vi "US fuel price.vi"() -> ()   [LabVIEW 2023]
doc: "Converts UK Fuel Prices to US fuel prices and vice versa"
panel:
  out "How much more expensive UK fuel is than US fuel":dbl=65.88302868943256 format="%#.1f %"
  out "How much cheaper US fuel is compared to UK fuel":dbl=63.12732642953957 format="%#.1g %"
  in  "stop":bool
  out "Price of UK Fuel converted to US units":dbl=7.079219668874475 format="$%02.2f/Gallon (US)"
  in  "Price of Fuel In US":dbl=3.39 format="$%02.2f/Gallon (US)"
  out "Price of US fuel converted to UK units":dbl=0.68956752697803 format="£%02.2f/Litre (UK)"
  in  "Dollar exchange rate":dbl=0.77 format="£%02.2f /$"
  in  "Price of Fuel In UK":dbl=1.44 format="£%02.2f/Litre (UK)"
  # "US-UK Fuel Price Convertor"
  # "Instructions\n1) Look up US dollar exchange rate (https://www.xe.com/en-gb/currencyconverter/convert/?Amount=1&From=USD&To=GBP) and update\n\n2) Look up UK fuel price (https://www.rac.co.uk/drive/advice/fuel-watch/) and update\n\n3) Look up US fuel price (https://gasprices.aaa.com/) and update\n\n4) Observe calculated values"
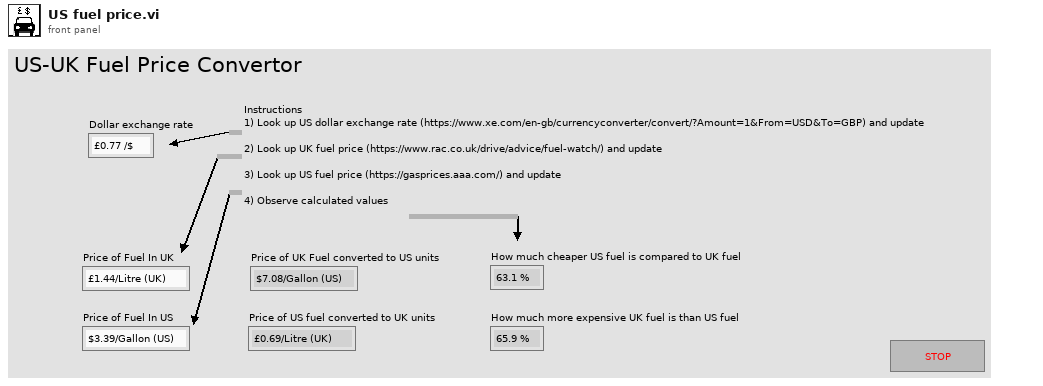
[diagram p1: front panel]
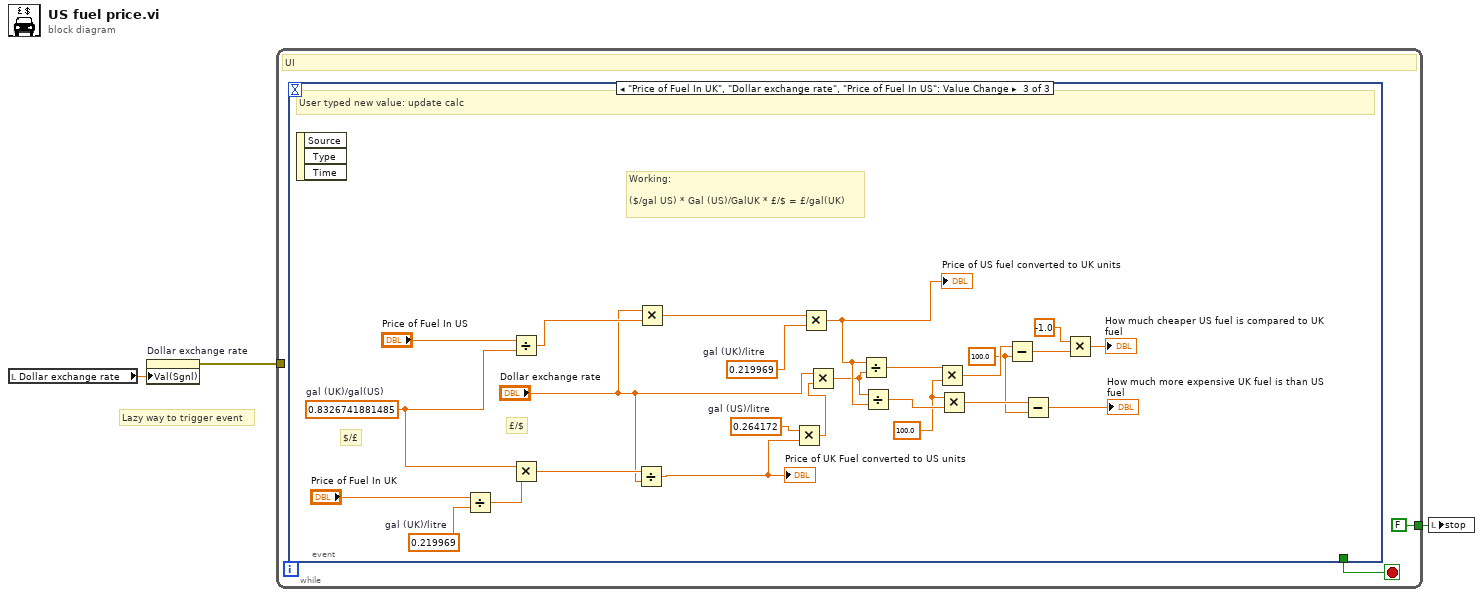
[diagram p0: block diagram]
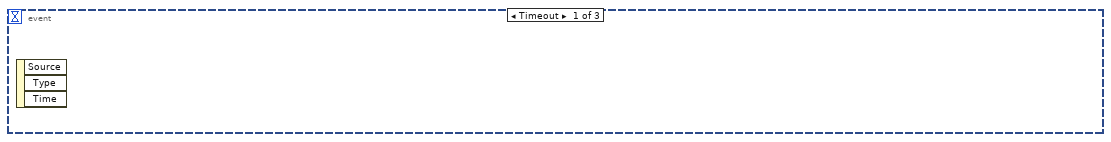
[diagram p2: hidden frame]
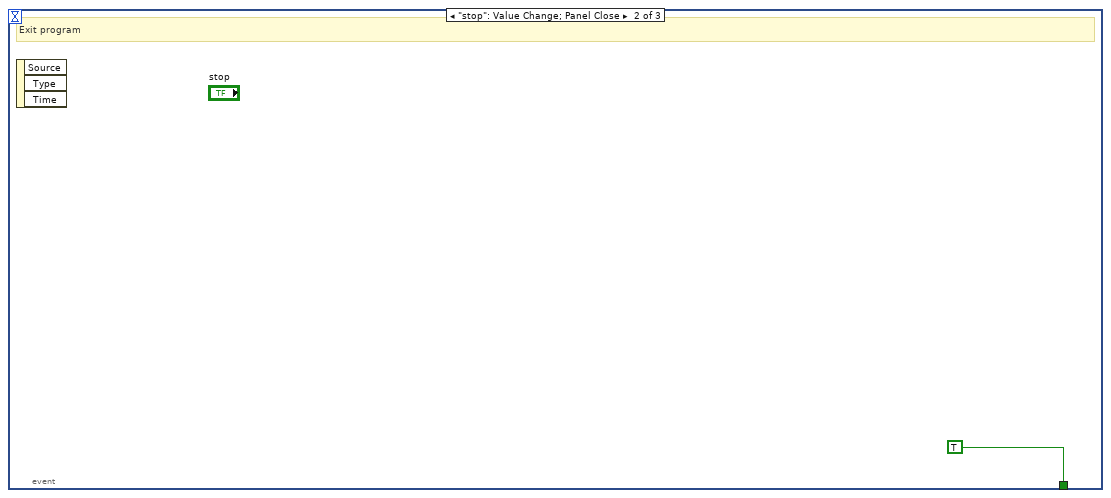
[diagram p3: hidden frame]
diagram:
  # "Lazy way to trigger event"
  n1 = local read "Dollar exchange rate"() -> (w2:dbl)
  n2 = property on="Dollar exchange rate" class="DigNum (strict)"("Val(Sgnl)"=w2) -> (error out=w1:errorcluster)  [unwired: 2 in, 1 out]
  n3 = while {
    tunnel: [FALSE ("stop")] -> w3
    tunnel: w1 -> [_]
    stop <- w5 stop-if-true
    # "UI"
    n4 = event shown="[2] \"Price of Fuel In UK\", \"Dollar exchange rate\", \"Price of Fuel In US\": Value Change" {
      selector: _ -> [_ _ _]
      dyn-events: _ -> [_ _ _]
      timeout: _ -> [_ _ _]
      tunnel: [_ TRUE _] -> w5
      event Timeout {
        n5 = event-data() -> ()  [unwired: 1 in, 3 out]
      }
      event "stop": Value Change; Panel Close {
        # "Exit program"
        n6 = event-data() -> ()  [unwired: 1 in, 3 out]
      }
      event "Price of Fuel In UK", "Dollar exchange rate", "Price of Fuel In US": Value Change {
        w15 = 100.0 ("y")
        w14 = 100.0 ("y")
        w13 = 0.264172  # gal (US)/litre
        w12 = 0.219969  # gal (UK)/litre
        w11 = 0.219969  # gal (UK)/litre
        w10 = 0.8326741881485  # gal (UK)/gal(US)
        # "Working:\n\n($/gal US) * Gal (US)/GalUK * £/$ = £/gal(UK)"
        # "£/$"
        # "$/£"
        # "User typed new value: update calc"
        n7 = event-data() -> ()  [unwired: 1 in, 3 out]
        n8 = Divide(x="Price of Fuel In UK", y=w12) -> (x/y=w22:dbl)
        n9 = Divide(x="Price of Fuel In US", y=w10) -> (x/y=w19:dbl)
        n10 = Multiply(x=w10, y=w22) -> (x*y=w18:dbl)
        n11 = Divide(x=w18, y="Dollar exchange rate") -> (x/y=w23:dbl)
        "Price of UK Fuel converted to US units" <- w23
        n12 = Multiply(x="Dollar exchange rate", y=w19) -> (x*y=w20:dbl)
        n13 = Multiply(x=w13, y=w23) -> (x*y=w9:dbl)
        n14 = Multiply(x=w20, y=w11) -> (x*y=w24:dbl)
        "Price of US fuel converted to UK units" <- w24
        n15 = Multiply(x="Dollar exchange rate", y=w9) -> (x*y=w7:dbl)
        n16 = Divide(x=w24, y=w7) -> (x/y=w25:dbl)
        n17 = Divide(x=w7, y=w24) -> (x/y=w26:dbl)
        n18 = Multiply(x=w25, y=w14) -> (x*y=w27:dbl)
        n19 = Multiply(x=w14, y=w26) -> (x*y=w28:dbl)
        n20 = Subtract(x=w27, y=w15) -> (x-y=w30:dbl)
        n21 = Subtract(x=w28, y=w15) -> (x-y=→"How much more expensive UK fuel is than US fuel":dbl)
        n22 = Multiply(x=-1.0, y=w30) -> (x*y=→"How much cheaper US fuel is compared to UK fuel":dbl)
      }
    }
  }
  n23 = local write "stop"(w3) -> ()
